vi "Init_DAQ_tasks.vi"(6 "error in":errorcluster, 9 "Parameter cluster":T3={"Acquisition parameters"={"Physical channels"="", "Shutter line"="", "Clock source"=0, "Triggered?"=FALSE, "Sample rate"=0.0, "Pixels to integrate"=0, "Effective data rate"=0.0, "Read chunk size"=0, "Samples to read"=0, "Run mode"=enum."Continuously"}, "Stimulation parameters"={"Physical channel"="", "Write chunk size"=0, "Sample rate"=0.0, "Stim onset"=0.0, "Stim frequency"=40.0, "ON time"=120.0, "OFF time"=1.0, "Repetitions"=1.0}} {"Acquisition parameters"."Pixels to integrate" min=1 step=1; "Acquisition parameters"."Sample rate" min=10.0 max=25000.0; "Acquisition parameters"."Clock source" items=["OnboardClock", "ExternalClock", "NoClock"]; "Stimulation parameters"."Write chunk size" min=100 max=100000; "Stimulation parameters"."Sample rate" min=10.0 max=10000.0; "Stimulation parameters"."Repetitions" min=0.0 max=10.0 step=1.0; "Stimulation parameters"."OFF time" min=0.0 max=1000.0; "Stimulation parameters"."ON time" min=0.0 max=1000.0; "Stimulation parameters"."Stim onset" min=0.0 max=100.0; "Stimulation parameters"."Stim frequency" min=1.0 max=40.0 step=1.0}) -> (0 "error out":errorcluster, 3 "Acq task out":refnum<k24>)   [LabVIEW 2010]
uses:
  C:/Program Files (x86)/National Instruments/LabVIEW 2010/vi.lib/ULx/ULx_LV.dll
  Program Files (x86)/National Instruments/LabVIEW 2010/vi.lib/ULx/ULx_LV.dll
  typedefs/acquisition_parameters_cluster.ctl
  typedefs/stimulation_parameters.ctl
  <vilib>/ULx/Create Channel.llb/ULx Create Channel (AI-Voltage-Basic).vi
  <vilib>/ULx/Timing.llb/ULx Timing (Sample Clock).vi
  <vilib>/ULx/Trigger.llb/ULx Basic Trigger (None).vi
  <vilib>/ULx/Trigger.llb/ULx Composite Trigger Start (ExtTTL).vi
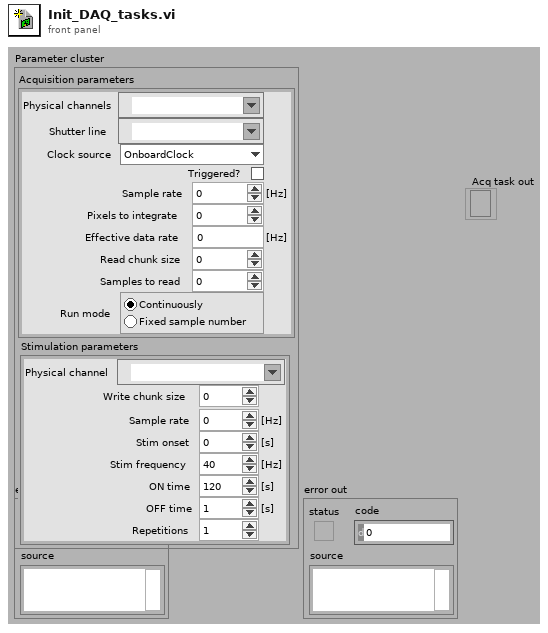
[diagram p1: front panel]
types:
  T1 = typedef "acquisition_parameters_cluster.ctl" = cluster{"Physical channels":refnum<k21>, "Shutter line":refnum<k21>, "Clock source":i32, "Triggered?":bool, "Sample rate":dbl, "Pixels to integrate":i32, "Effective data rate":dbl, "Read chunk size":i32, "Samples to read":i32, "Run mode":enum32{"Continuously", "Fixed sample number"}}
  T2 = typedef "stimulation_parameters.ctl" = cluster{"Physical channel":tag, "Write chunk size":i32, "Sample rate":dbl, "Stim onset":dbl, "Stim frequency":dbl, "ON time":dbl, "OFF time":dbl, "Repetitions":dbl}
  T3 = cluster{"Acquisition parameters":T1, "Stimulation parameters":T2}
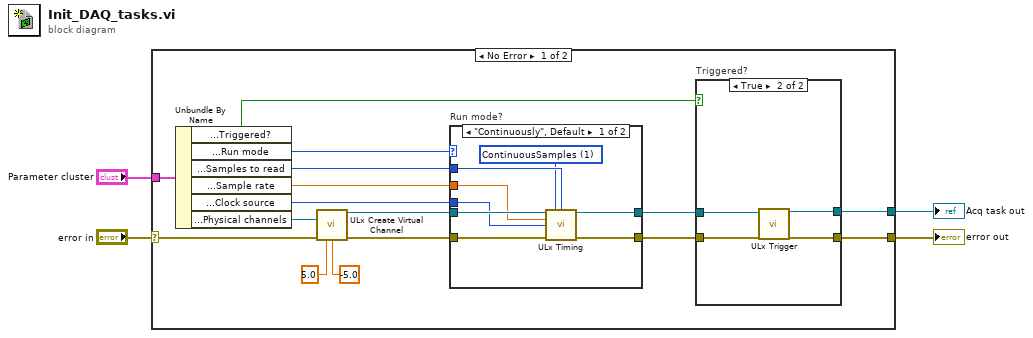
[diagram p0: block diagram]
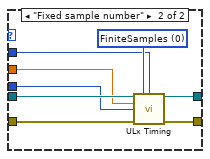
[diagram p2: hidden frame]
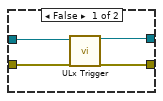
[diagram p3: hidden frame]
diagram:
  n1 = case shown="No Error" "error in" {
    selector: "error in" -> [w6 w45]
    tunnel: [w20 _] -> w4
    tunnel: [w5 w45] -> w3
    tunnel: "Parameter cluster" -> [w7 _]
    frame No Error {
      n2 = Unbundle By Name(w7) -> ("Acquisition parameters.Triggered?"=w10:bool, "Acquisition parameters.Run mode"=w9:enum32{"Continuously", "Fixed sample number"}, "Acquisition parameters.Samples to read"=w8:i32, "Acquisition parameters.Sample rate"=w16:dbl, "Acquisition parameters.Clock source"=w15:i32, "Acquisition parameters.Physical channels"=w11:refnum<k21>)
      n3 = call-poly <vilib>:"ULx Create Virtual Channel.vi"("maximum value"=5.0, "minimum value"=-5.0, "physical channels"=w11, "error in"=w6) -> ("task out"=w17:refnum<k24>, "error out"=w14:errorcluster)  [unwired: 10 in]
      n4 = case "Run mode?" shown="\"Continuously\", Default" w9 {
        tunnel: [w25 w36] -> w19
        tunnel: [w27 w35] -> w18
        tunnel: w17 -> [w26 w33]
        tunnel: w16 -> [w23 w32]
        tunnel: w15 -> [w24 w31]
        tunnel: w14 -> [w28 w30]
        tunnel: w8 -> [w22 w29]
        frame "Continuously", Default {
          w21 = 1 items=["FiniteSamples", "ContinuousSamples"] ("sample mode")
          n5 = call-poly <vilib>:"ULx Timing.vi"("task in"=w26, "sample mode"=w21, "samples per channel"=w22, "rate"=w23, "clock source"=w24, "error in"=w28) -> ("task out"=w25:refnum<k24>, "error out"=w27:errorcluster)  [unwired: 8 in]
        }
        frame "Fixed sample number" {
          w34 = 0 items=["FiniteSamples", "ContinuousSamples"] ("sample mode")
          n6 = call-poly <vilib>:"ULx Timing.vi"("task in"=w33, "sample mode"=w34, "samples per channel"=w29, "rate"=w32, "clock source"=w31, "error in"=w30) -> ("task out"=w36:refnum<k24>, "error out"=w35:errorcluster)  [unwired: 8 in]
        }
      }
      n7 = case "Triggered?" shown="True" w10 {
        tunnel: w18 -> [w39 w44]
        tunnel: [w37 w43] -> w5
        tunnel: w19 -> [w40 w42]
        tunnel: [w38 w41] -> w20
        frame False {
          n8 = call-poly <vilib>:"ULx Trigger.vi"("task in"=w40, "error in"=w39) -> ("task out"=w38:refnum<k24>, "error out"=w37:errorcluster)  [unwired: 16 in]
        }
        frame True {
          n9 = call-poly <vilib>:"ULx Trigger.vi"("task in"=w42, "error in"=w44) -> ("task out"=w41:refnum<k24>, "error out"=w43:errorcluster)  [unwired: 16 in]
        }
      }
    }
    frame Error {
    }
  }
  "Acq task out" <- w4
  "error out" <- w3
